vi "sensor.vi"(11 "计次读取":i32) -> (1 "计次输出":dbl, 2 "传感器端口":dynamicdata(graph), 3 "传感器端口平均值":dbl)   [LabVIEW 2018]
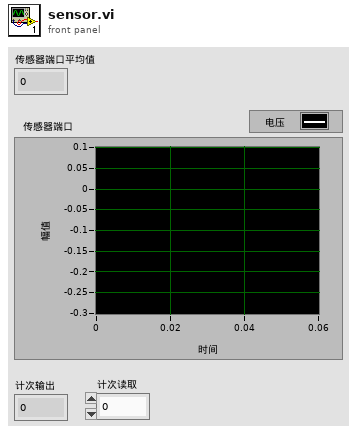
[diagram p1: front panel]
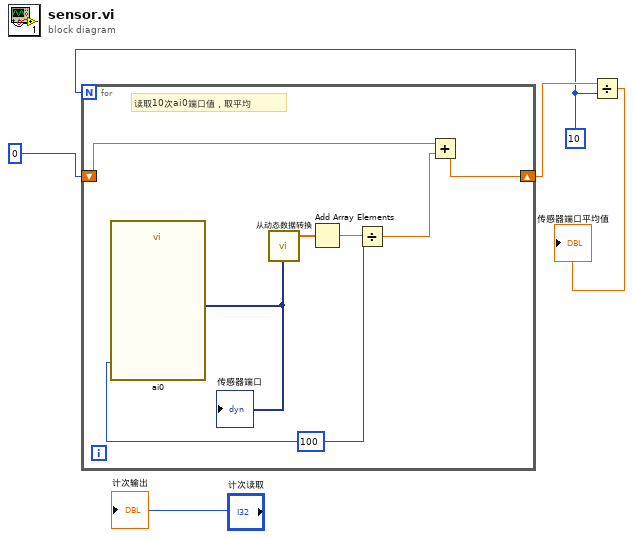
[diagram p0: block diagram]
diagram:
  w3 = 10
  n1 = for {
    N: w3 -> [_]
    shift-right: [w12] -> w4
    shift-left: 0 -> [w11]
    w8 = 100
    # "读取10次ai0端口值，取平均"
    n2 = call "ai0"("采样数"=w8) -> ("data"=w10:dynamicdata)  [unwired: 16 in, 2 out]
    "传感器端口" <- w10
    n3 = call "从动态数据转换"("Dynamic Data Type"=w10) -> ("Array"=w9:dbl[])  [unwired: 3 in]
    n4 = Add Array Elements(numeric array=w9) -> (sum=w7:dbl)
    n5 = Divide(x=w7, y=w8) -> (x/y=w6:dbl)
    n6 = Add(x=w11, y=w6) -> (x+y=w12:dbl)
  }
  n7 = Divide(x=w4, y=w3) -> (x/y=→"传感器端口平均值":dbl)
  "计次输出" <- "计次读取"
